vi "Query with 2D Double Result.vi"(8 "error in (no error)":errorcluster, 10 "Query string":string, 11 "mysql in":refnum<class "mysql.lvclass">) -> (0 "error out":errorcluster, 2 "Result":dbl[][](array[numeric]), 3 "mysql out":refnum<class "mysql.lvclass">)   [LabVIEW 2020, in "mysql.lvlib" / "mysql.lvclass"]
uses:
  mysql.lvclass
  d5d65c61-9ad0-4acb-b6d0-7193bdbe97b3.vi
  d5d65c61-9ad0-4acb-b6d0-7193bdbe97b3.vi/f50bcc16-7a1d-4020-a60d-000cbe5ba8c9.vi
  d5d65c61-9ad0-4acb-b6d0-7193bdbe97b3.vi/c3d2ca68-206d-4d6e-bef5-c06e852db6ed.vi
  private/Mysql command.vi
  private/Mysql data reader 2D double.vi
  private/ping connection and reopen if needed.vi
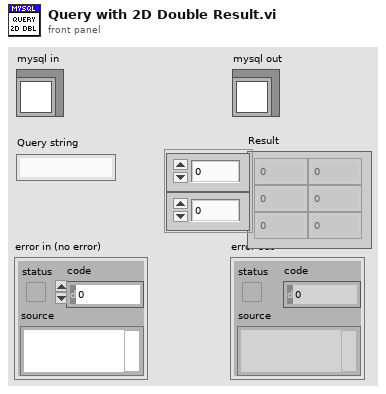
[diagram p1: front panel]
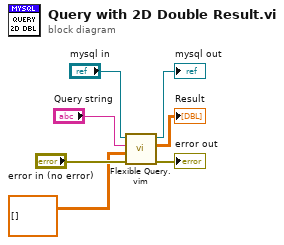
[diagram p0: block diagram]
diagram:
  n1 = call "Flexible Query.vim"("error in (no error)"="error in (no error)", "Type in"=dbl[][] [] ("Result 2"), "Query string"="Query string", "mysql in"="mysql in") -> ("error out"=→"error out":errorcluster, "Result"=→"Result":dbl[][], "mysql out"=→"mysql out":refnum<class "mysql.lvclass">)  [unwired: 5 in]
